vi "InitializeTachometerState.vi"(8 "error in (no error)":errorcluster, 11 "Tachometer in":T1) -> (0 "error out":errorcluster, 3 "Tachometer out":T1)   [LabVIEW 2017, in "CmsVirtualChannel.lvlib"]
uses:
  <vilib>/addons/InsightCM/Devices/Shared/Cms/CmsVirtualChannel/CmsVirtualChannel.lvlib
  <vilib>/addons/InsightCM/Devices/Shared/Cms/CmsVirtualChannel/controls/Tachometer.ctl
  <vilib>/addons/InsightCM/Utilities/Analysis/Vibration/controls/Tachometer.ctl
  <vilib>/addons/InsightCM/Utilities/Analysis/Vibration/controls/DigitalTachometer.ctl
  <vilib>/addons/InsightCM/Utilities/Analysis/Vibration/VibrationAnalysisFunctions.lvlib
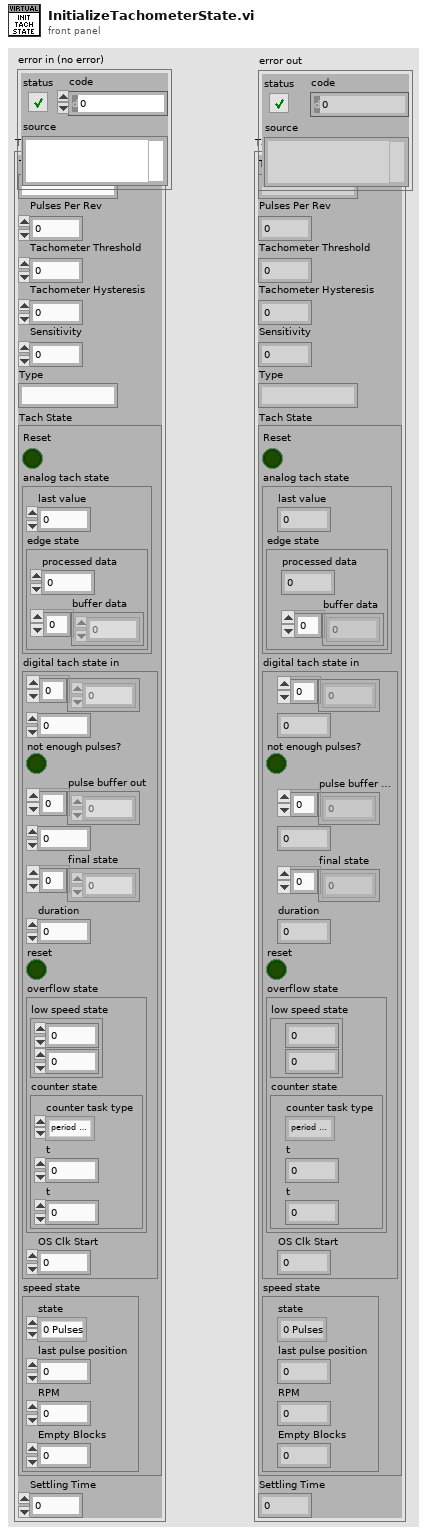
[diagram p1: front panel]
types:
  T1 = typedef "CmsVirtualChannel.lvlib/Tachometer.ctl" = cluster{"Tachometer Slope":string, "Pulses Per Rev":i32, "Tachometer Threshold":dbl, "Tachometer Hysteresis":dbl, "Sensitivity":dbl, "Type":string, "Tach State":T2, "Settling Time":dbl}
  T2 = typedef "VibrationAnalysisFunctions.lvlib/Tachometer.ctl" = cluster{"Reset":bool, "analog tach state":cluster{"last value":dbl, "edge state":cluster{"processed data":dbl, "buffer data":dbl[]}}, "digital tach state in":T3, "speed state":cluster{"state":enum16{"0 Pulses", "1 Pulse", "2+ Pulses"}, "last pulse position":dbl, "RPM":dbl, "Empty Blocks":i32}}
  T3 = typedef "VibrationAnalysisFunctions.lvlib/DigitalTachometer.ctl" = cluster{dbl[], i32, "not enough pulses?":bool, "pulse buffer out":dbl[], i32, "final state":dbl[], "duration":dbl, "reset":bool, "overflow state":cluster{"low speed state":cluster{dbl, ext}, "counter state":cluster{"counter task type":enum16{"period measurement", "event counting"}, "t":dbl, "t":dbl}}, "OS Clk Start":dbl}
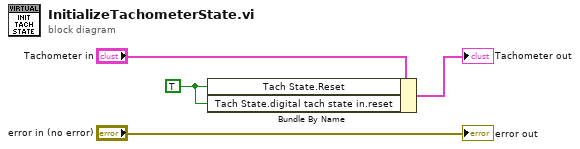
[diagram p0: block diagram]
diagram:
  w2 = TRUE ("Reset")
  n1 = Bundle By Name(cluster="Tachometer in", "Tach State.Reset"=w2, "Tach State.digital tach state in.reset"=w2) -> (→"Tachometer out":T1)
  "error out" <- "error in (no error)"
